vi "proportional integral derivative.vi"() -> ()   [LabVIEW 2020]
uses:
  <vilib>/addons/control/pid/NI_PID_pid.lvlib
  <vilib>/addons/control/pid/pid.llb/PID Advanced (DBL).vi
panel:
  in  "SP":dbl(slide) scale=0.0..100.0
  out "PV(output)":dbl(slide) scale=0.0..100.0
  out "?":dbl(knob) scale=0.0..100.0 scale format="%#_3g"
  in  "stop":bool
  out "Waveform Chart":cluster{"LCV":dbl, "SP":dbl, "Plant Output":dbl}(graph)
  in  "process parameters":T1={"static gain"=2.5, "lag (s)"=2.5, "deadtime (s)"=0.001, "load"=0.0, "deadband"=0.0, "sensor noise"=0.0, "initial PV"=30.0, "plant noise"=0.0} {"plant noise" format="%.2f"; "initial PV" format="%.2f"; "sensor noise" format="%.2f"; "lag (s)" format="%.2f"; "deadtime (s)" format="%.2f"; "deadband" format="%.1f"; "load" format="%.2f"; "static gain" format="%.2f"}
  in  "PID gains":T2={"proportional gain (Kc)"=1.0, "integral time (Ti, min)"=0.01, "derivative time (Td, min)"=0.0} {"derivative time (Td, min)" format="%.3f"; "integral time (Ti, min)" format="%.3f"; "proportional gain (Kc)" format="%.3f"}
  in  "auto? (T)":bool=TRUE
  in  "LCV":dbl format="%.2f"
  # "LCV"
  # "LT"
  # "Liquid in"
  # "Liquid out"
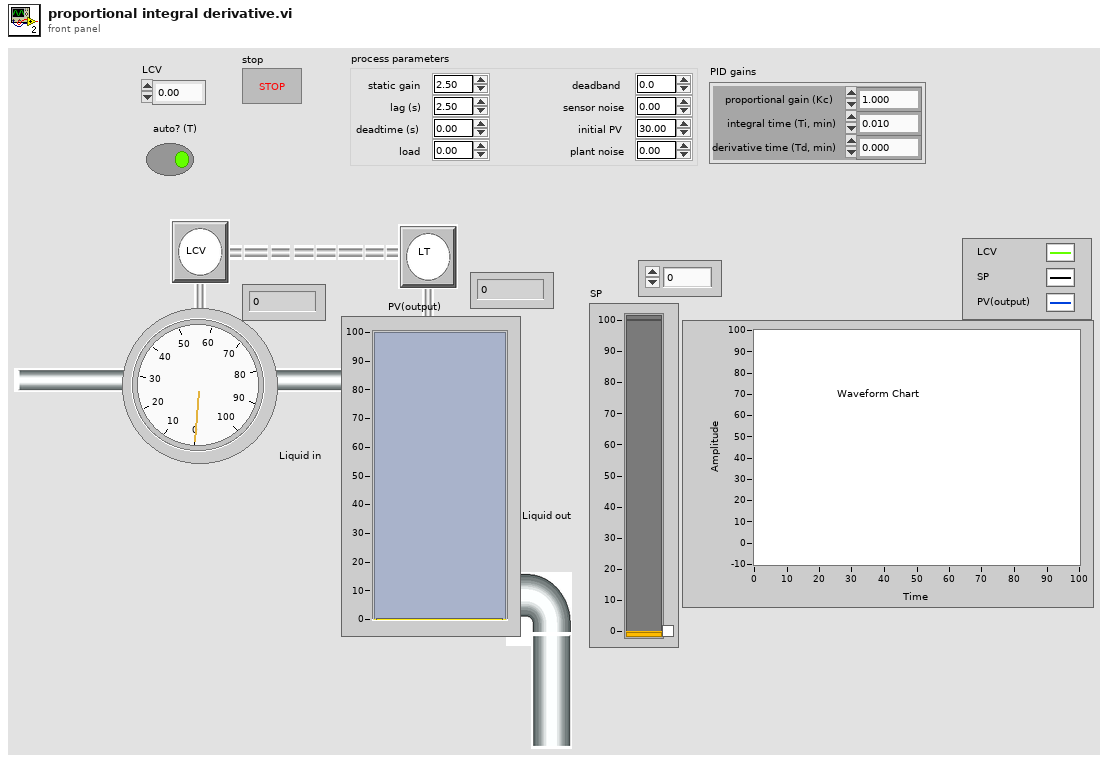
[diagram p1: front panel]
types:
  T1 = cluster{"static gain":dbl, "lag (s)":dbl, "deadtime (s)":dbl, "load":dbl, "deadband":dbl, "sensor noise":dbl, "initial PV":dbl, "plant noise":dbl}
  T2 = cluster{"proportional gain (Kc)":dbl, "integral time (Ti, min)":dbl, "derivative time (Td, min)":dbl}
  T3 = cluster{"output":dbl, "SP":dbl, "Plant Output":dbl}
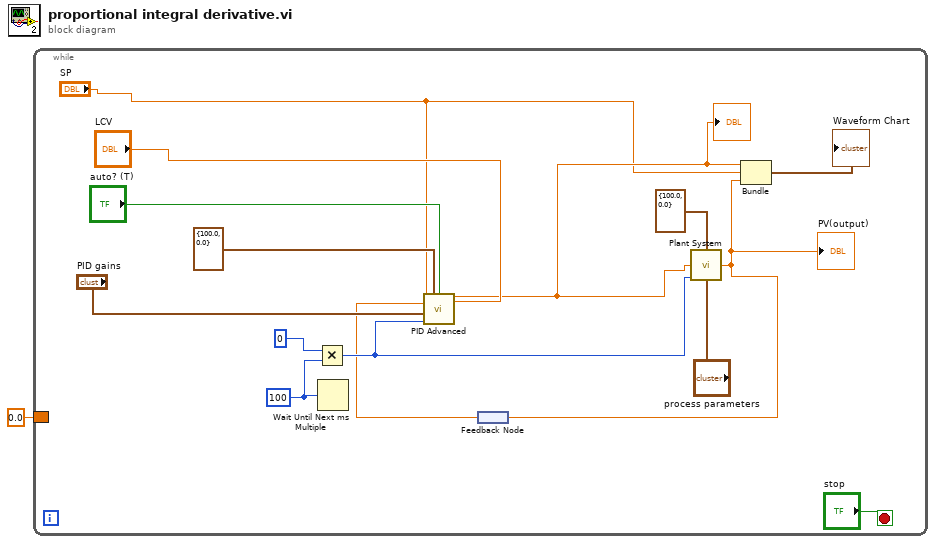
[diagram p0: block diagram]
diagram:
  n1 = while {
    border: 0.0 ("Plant Output") -> [_]
    stop <- "stop" stop-if-true
    w8 = u32 100 ("millisecond multiple")
    n2 = Multiply(x=u32 0, y=w8) -> (x*y=w7:u32)
    n3 = Wait Until Next ms Multiple(millisecond multiple=w8) -> ()  [unwired: 1 out]
    n4 = feedback #1() -> (w6:dbl)
    n5 = call-poly <vilib>:"PID Advanced.vi"("setpoint"="SP", "output range"=cluster{"output high":dbl, "output low":dbl} {"output high"=100.0, "output low"=0.0}, "auto? (T)"="auto? (T)", "manual control"="LCV", "process variable"=w6, "PID gains"="PID gains", "dt (s)"=w7) -> ("output"=w4:dbl)  [unwired: 7 in, 1 out]
    "?" <- w4
    n6 = call "Plant System.vi"("output saturation range"=cluster{"output high":dbl, "output low":dbl} {"output high"=100.0, "output low"=0.0}, "Plant Input"=w4, "dt (s)"=w7, "process parameters"="process parameters") -> ("Plant Output"=w3:dbl)  [unwired: 11 in]
    "PV(output)" <- w3
    n7 = feedback-in #1(w3) -> ()
    n8 = Bundle("output"=w4, "SP"="SP", "Plant Output"=w3) -> (→"Waveform Chart":T3)  [unwired: 1 in]
  }
